vi "OCR Training Tool.vi"() -> ()   [LabVIEW 2018, in "Receipt Parsing.lvlib"]
uses:
  Receipt Parsing.lvlib
  <vilib>/vision/OCR.llb/IMAQ OCR Character Report 2.ctl
  <vilib>/vision/NI_Vision_Development_Module.lvlib
panel:
  out "spreadsheet string":string
  out "Number of Objects":i32
  out "Image 2":T1(plugin-control)
  in  "Min height":i32=450
  out "height (pixels)":i32
  out "width (pixels)":i32
  in  "Submit":bool
  in  "Skip":bool
  in  "Quit":bool
  in  "Character":string
  in  "Min classification score":i32=450
  out "Read String":string
  out "Character Reports":T2[](array[typedef]) {"Character Statistics"."Threshold Range"."Upper value" format="%.2f"; "Character Statistics"."Threshold Range"."Lower value" format="%.2f"}
  out "selected path":path
  out "Post-trained Read":string
  out "Pre-trained Read":string
  out "Image":T1(plugin-control)
  # "Overview: Demonstrates how to train characters to an OCR and compare the readings. \nRequirements: LabVIEW Base Development System 2012 (or compatible)\n                             NI Vision Development Module 2012 (or compatible)\nInstructions: \n1. Run the VI."
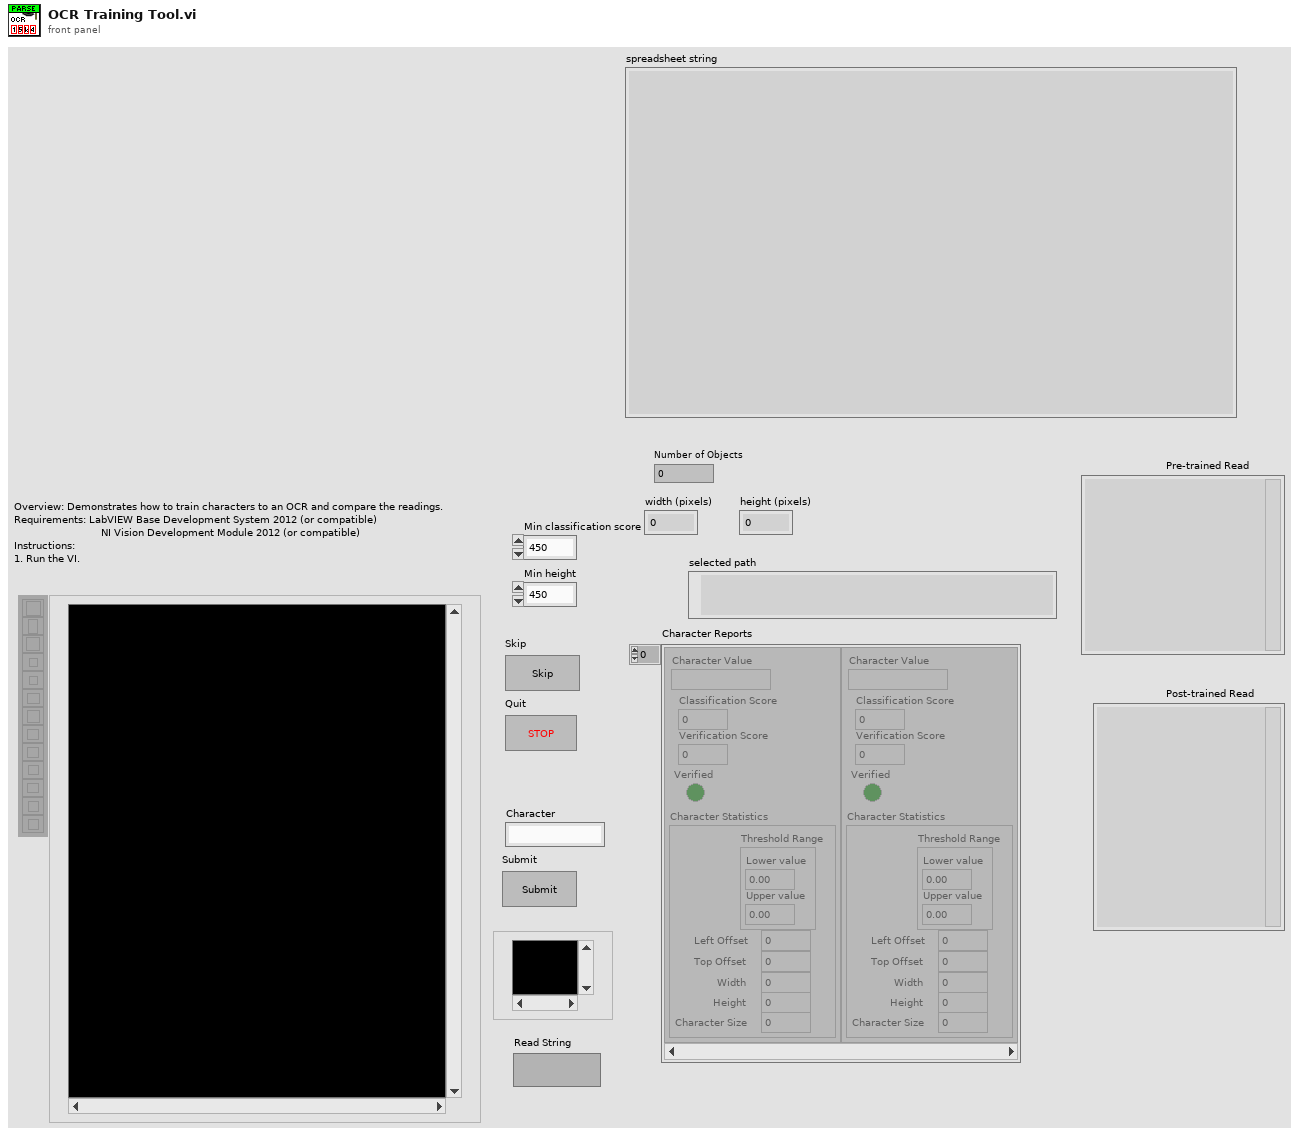
[diagram p1: front panel]
types:
  T1 = typedef "IMAQ Image.ctl" = refnum<image>
  T2 = typedef "IMAQ OCR Character Report 2.ctl" = cluster{"Character Value":string, "Classification Score":i32, "Verification Score":i32, "Verified":bool, "Character Statistics":cluster{"Threshold Range":cluster{"Lower value":sgl, "Upper value":sgl}, "Left Offset":i32, "Top Offset":i32, "Width":i32, "Height":i32, "Character Size":i32}}
  T3 = cluster{"Objects":u16, "Threshold":i32, "Reject Border":bool, "Fill Holes":bool, "Min Object Size":bool, "Min Size":i32, "Max Object Size":bool, "Max Size":i32, "Show Search Area":bool, "Show Center":bool, "Show Bounding Box":bool}
  T4 = typedef "IMAQ OCR Session.ctl" = refnum<k1>
  T5 = typedef "IMAQ Rectangle" = cluster{"Left":i32, "Top":i32, "Right":i32, "Bottom":i32, "Rotation":dbl}
  T6 = cluster{"Object Center":cluster{"X":sgl, "Y":sgl}, "Bounding Box":cluster{"X Left":i32, "Y Top":i32, "X Right":i32, "Y Bottom":i32}, "Area":sgl, "Orientation":sgl, "Aspect Ratio":sgl, "Nb Holes":i32}[]
  T7 = cluster{"X Left":i32, "Y Top":i32, "X Right":i32, "Y Bottom":i32}
  T8 = typedef "ROI Descriptor" = cluster{"Global Rectangle":i32[], "Contours":cluster{"ID":enum32{"External", "Internal"}, "Type":u32, "Coordinates":i32[]}[]}
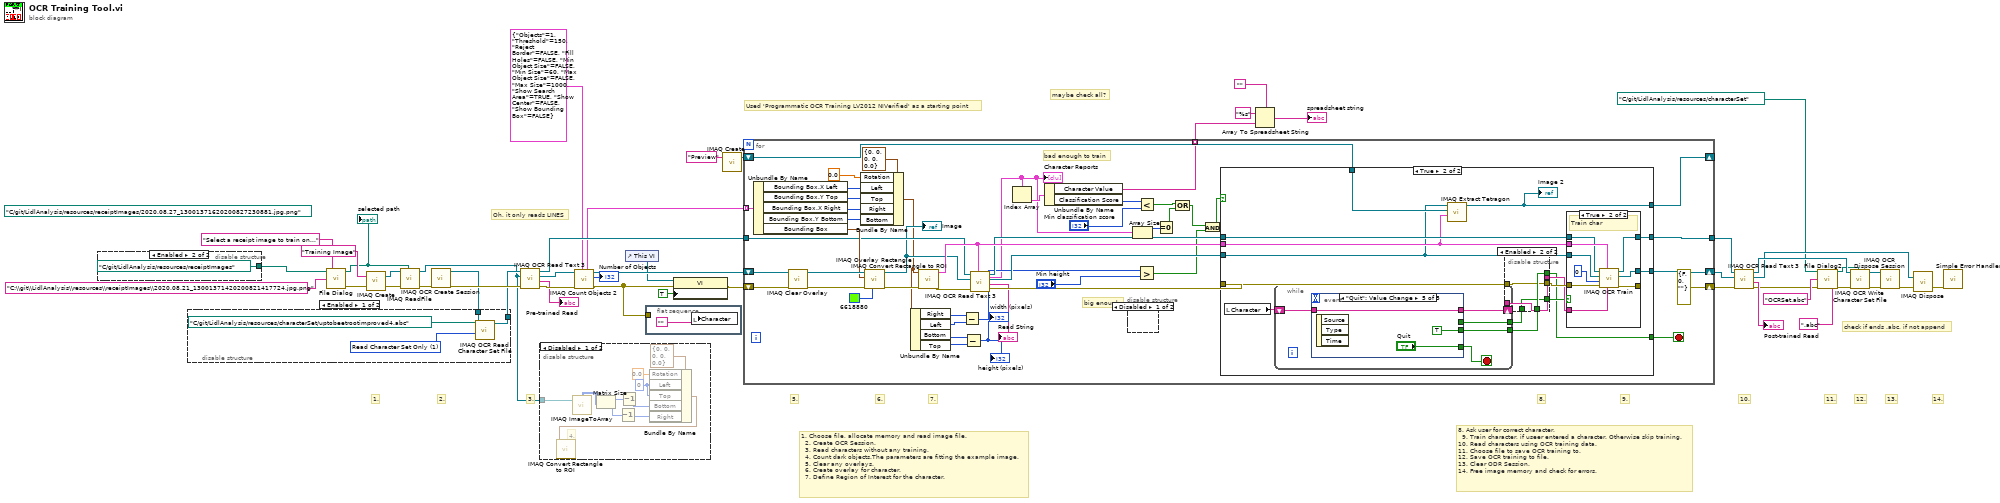
[diagram p0: block diagram]
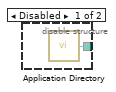
[diagram p3: hidden frame]
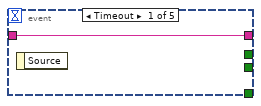
[diagram p7: hidden frame]
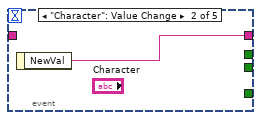
[diagram p8: hidden frame]
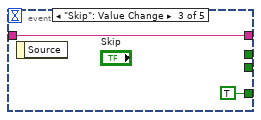
[diagram p9: hidden frame]
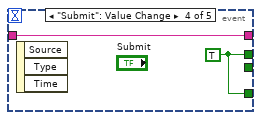
[diagram p10: hidden frame]
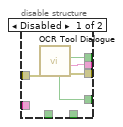
[diagram p11: hidden frame]
diagram:
  (unwired) path "C:/git/LidlAnalysis/resources/receiptImages/2020.08.27_13001371620200827230881.jpg.png" ("File Path")
  # "Oh, it only reads LINES"
  # "maybe check all?"
  # "check if ends .abc, if not append"
  # "Used 'Programmatic OCR Training LV2012 NIVerified' as a starting point"
  # "8. Ask user for correct character.\n  9. Train character, if useer entered a character. Otherwise skip training.\n10. Read characters using OCR training data.\n11. Choose file to save OCR training to.\n12. Save OCR training to file.\n13. Clear ODR Session.\n14. Free image memory and check for errors."
  # "1. Choose file, allocate memory and read image file.\n  2. Create OCR Session.\n  3. Read characters without any training.\n  4. Count dark objects.The parameters are fitting the example image.\n  5. Clear any overlays.\n  6. Create overlay for character.\n  7. Define Region of Interest for the character."
  # "14."
  # "13."
  # "12."
  # "11."
  # "10."
  # "9."
  # "8."
  # "7."
  # "6."
  # "5."
  # "3."
  # "2."
  # "1."
  n1 = disable-structure shown="Enabled" {
    disable-tunnel: [w48 path "C:/git/LidlAnalysis/resources/receiptImages" ("start path")] -> w29
    frame Disabled {
      n2 = call <vilib>:"Application Directory.vi"() -> ("Application Directory"=w48:path)
    }
    frame Enabled {
    }
  }
  n3 = call "File Dialog"("start path"=w29, "prompt"="Select a receipt image to train on...", "default name"="C:\\git\\LidlAnalysis\\resources\\receiptImages\\2020.08.21_13001371420200821417724.jpg.png") -> ("selected path"=w26:path, "error out"=w27:errorcluster)  [unwired: 9 in, 2 out]
  "selected path" <- w26
  n4 = call "IMAQ Create"("Image Name"="Training Image", "error in (no error)"=w27) -> ("New Image"=w46:T1, "error out"=w44:errorcluster)  [unwired: 3 in]
  n5 = call "IMAQ ReadFile"("File Path"=w26, "error in (no error)"=w44, "Image"=w46) -> ("error out"=w43:errorcluster, "Image Out"=w10:T1)  [unwired: 4 in, 3 out]
  n6 = call "IMAQ OCR Create Session"("error in (no error)"=w43) -> ("error out"=w39:errorcluster, "IMAQ OCR Session"=w20:T4)  [unwired: 9 in]
  n7 = disable-structure shown="Enabled" {
    disable-tunnel: w20 -> [w52 w54]
    disable-tunnel: [w51 w54] -> w19
    frame Enabled {
      w53 = 1 items=["Read All", "Read Character Set Only", "Read Properties Only"] ("Read Options")
      n8 = call "IMAQ OCR Read Character Set File"("File Path"=path "C:/git/LidlAnalysis/resources/characterSet/uptobeetrootimproved4.abc", "Read Options"=w53, "IMAQ OCR Session"=w52) -> ("IMAQ OCR Session (dup)"=w51:T4)  [unwired: 6 in, 2 out]
    }
    frame Disabled {
    }
  }
  n9 = call "IMAQ OCR Read Text 3"("error in (no error)"=w39, "Image"=w10, "IMAQ OCR Session"=w19) -> ("error out"=w47:errorcluster, "Read String"=→"Pre-trained Read":string, "Image (dup)"=w11:T1, "IMAQ OCR Session (dup)"=w40:T4)  [unwired: 3 in, 2 out]
  n10 = disable-structure shown="Disabled" {
    disable-tunnel: w10 -> [w60 _]
    frame Disabled {
      w62 = 0 ("Left")
      # "4."
      n11 = call "IMAQ ImageToArray"("Image"=w60) -> ("Image Pixels (U8)"=w64:u8[][])  [unwired: 3 in, 4 out]
      n12 = Matrix Size(0:w64) -> (1:w58:i32, 2:w55:i32)
      n13 = Decrement(x=w55) -> (x-1=w56:i32)
      n14 = Decrement(x=w58) -> (x-1=w57:i32)
      n15 = Bundle By Name(cluster=T5 {"Left"=0, "Top"=0, "Right"=0, "Bottom"=0, "Rotation"=0.0} ("Rectangle"), "Rotation"=0.0, "Left"=w62, "Top"=w62, "Bottom"=w57, "Right"=w56) -> (w61:T5)
      n16 = call "IMAQ Convert Rectangle to ROI"("Rectangle"=w61) -> ()  [unwired: 8 in, 2 out]
    }
    frame Enabled {
    }
  }
  n17 = call "IMAQ Count Objects 2"("Settings"=T3 {"Objects"=1, "Threshold"=150, "Reject Border"=FALSE, "Fill Holes"=FALSE, "Min Object Size"=FALSE, "Min Size"=60, "Max Object Size"=FALSE, "Max Size"=1000, "Show Search Area"=TRUE, "Show Center"=FALSE, "Show Bounding Box"=FALSE}, "error in (no error)"=w47, "Image"=w11) -> ("error out"=w1:errorcluster, "Number of Objects"=→"Number of Objects":i32, "Image Out"=w34:T1, "Objects"=w33:T6)  [unwired: 4 in, 1 out]
  n18 = control-ref of="This VI"() -> (w14:refnum<vi>)
  n19 = flat-sequence {
    tunnel: w1 -> [_]
    frame #0 {
      n20 = local write "Character"("") -> ()
    }
  }
  n21 = property class="VI"(reference=w14, error in=w1, "Front Panel.IsFrontmost"=TRUE ("Front Panel Window:Is Frontmost")) -> (error out=w13:errorcluster)  [unwired: 1 out]
  n22 = call "IMAQ Create"("Image Name"="Preview") -> ("New Image"=w8:T1)  [unwired: 4 in, 1 out]
  n23 = for {
    shift-right: [errorcluster {"status"=FALSE, "code"=0, "source"=""} ("error out")] -> w35
    shift-left: w13 -> [w112]
    shift-right: [w111] -> w17
    shift-left: w34 -> [w108]
    tunnel: w33 -> [w106] mode=indexing
    tunnel: w40 -> [w90]
    tunnel: [w110] -> w18
    shift-right: [w74] -> _
    shift-left: w8 -> [w73]
    tunnel: [w66] -> w5 mode=indexing
    stop <- w95 stop-if-true
    # "bad enough to train"
    # "big enough"
    n24 = Unbundle By Name(w106) -> ("Bounding Box.X Left"=w101:i32, "Bounding Box.Y Top"=w100:i32, "Bounding Box.X Right"=w99:i32, "Bounding Box.Y Bottom"=w98:i32, "Bounding Box"=w105:T7)
    n25 = call "IMAQ Clear Overlay"("error in (no error)"=w112, "Image"=w108) -> ("error out"=w109:errorcluster, "Image Out"=w107:T1)  [unwired: 8 in]
    n26 = Bundle By Name(cluster=T5 {"Left"=0, "Top"=0, "Right"=0, "Bottom"=0, "Rotation"=0.0} ("Rectangle"), "Rotation"=0.0, "Left"=w101, "Top"=w100, "Right"=w99, "Bottom"=w98) -> (w83:T5)
    n27 = call "IMAQ Overlay Rectangle"("Color"=u32 6618880, "error in (no error)"=w109, "Rectangle"=w105, "Image"=w107) -> ("error out"=w103:errorcluster, "Image Out"=w89:T1)  [unwired: 6 in]
    "Image" <- w89
    n28 = Unbundle By Name(w83) -> ("Right"=w82:i32, "Left"=w81:i32, "Bottom"=w80:i32, "Top"=w79:i32)
    n29 = call "IMAQ Convert Rectangle to ROI"("error in (no error)"=w103, "Rectangle"=w83) -> ("error out"=w94:errorcluster, "ROI Descriptor"=w92:T8)  [unwired: 7 in]
    n30 = Subtract(x=w82, y=w81) -> (x-y=→"width (pixels)":i32)
    n31 = Subtract(x=w80, y=w79) -> (x-y=w75:i32)
    "height (pixels)" <- w75
    n32 = call "IMAQ OCR Read Text 3"("ROI Descriptor"=w92, "error in (no error)"=w94, "Image"=w89, "IMAQ OCR Session"=w90) -> ("error out"=w93:errorcluster, "Read String"=→"Read String":string, "Image (dup)"=w88:T1, "IMAQ OCR Session (dup)"=w91:T4, "Character Reports"=w72:T2[])  [unwired: 2 in, 1 out]
    "Character Reports" <- w72
    n33 = Index Array(array=w72) -> (element=w86:T2)  [unwired: 1 in]
    n34 = Unbundle By Name(w86) -> ("Character Value"=w66:string, "Classification Score"=w85:i32)
    n35 = disable-structure shown="Disabled" {
      frame Disabled {
      }
      frame Enabled {
      }
    }
    n36 = Array Size(array=w72) -> (size(s)=w71:i32)
    n37 = Greater?(x=w75, y="Min height") -> (0:w69:bool)
    n38 = Less?(x=w85, y="Min classification score") -> (x < y?=w77:bool)
    n39 = Equal To 0?(x=w71) -> (x = 0?=w70:bool)
    n40 = Compound Arithmetic op=OR(w77, w70) -> (w68:bool)
    n41 = And(x=w68, y=w69) -> (x .and. y?=w67:bool)
    n42 = case shown="True" w67 {
      tunnel: [w115 w131] -> w111
      tunnel: [w114 w130] -> w110
      tunnel: [_ w126] -> w95
      tunnel: w93 -> [_ w124]
      tunnel: w92 -> [_ w119]
      tunnel: w91 -> [w114 w125]
      tunnel: w88 -> [w115 w118]
      tunnel: w73 -> [w113 w120]
      tunnel: [w113 w117] -> w74
      frame False {
        # "No need to train"
      }
      frame True {
        n43 = local read "Character"() -> (w116:string)
        n44 = while {
          tunnel: [w135] -> w123
          tunnel: [w134] -> w121
          shift-right: [w133] -> w122
          shift-left: w116 -> [w132]
          stop <- w136 stop-if-true
          n45 = event shown="[4] \"Quit\": Value Change" {
            selector: _ -> [_ _ _ _ _]
            dyn-events: _ -> [_ _ _ _ _]
            timeout: _ -> [_ _ _ _ _]
            tunnel: [_ _ TRUE ("Quit") w142 "Quit"] -> w136
            tunnel: [_ _ _ _ TRUE] -> w135
            tunnel: [_ _ _ w142 _] -> w134
            tunnel: [w137 w138 w139 w141 w143] -> w133
            tunnel: w132 -> [w137 _ w139 w141 w143]
            event Timeout {
              n46 = event-data() -> ()  [unwired: 1 in, 1 out]
            }
            event "Character": Value Change {
              n47 = event-data() -> ("NewVal"=w138:string)  [unwired: 1 in]
            }
            event "Skip": Value Change {
              n48 = event-data() -> ()  [unwired: 1 in, 1 out]
            }
            event "Submit": Value Change {
              w142 = TRUE
              n49 = event-data() -> ()  [unwired: 1 in, 3 out]
            }
            event "Quit": Value Change {
              n50 = event-data() -> ()  [unwired: 1 in, 3 out]
            }
          }
        }
        n51 = call-poly "IMAQ Extract Tetragon"("ROI Descriptor"=w119, "Image Dst"=w120, "Image Src"=w118) -> ("Image Dst Out"=w117:T1)  [unwired: 7 in, 1 out]
        "Image 2" <- w117
        n52 = disable-structure shown="Enabled" {
          disable-tunnel: [w150 w152] -> w129
          disable-tunnel: [w149 w153] -> w128
          disable-tunnel: [w148 w151] -> w127
          disable-tunnel: w124 -> [w147 w152]
          disable-tunnel: [w146 w154] -> w126
          disable-tunnel: w123 -> [_ w154]
          disable-tunnel: w122 -> [_ w153]
          disable-tunnel: w121 -> [_ w151]
          frame Disabled {
            n53 = call "OCR Tool Dialogue.vi"("error in (no error)"=w147) -> ("error out"=w150:errorcluster, "Character"=w149:string, "Quitted?"=w146:bool, "Enter Char"=w148:bool)  [unwired: 7 in]
          }
          frame Enabled {
          }
        }
        n54 = case shown="True" w127 {
          tunnel: [w156 w165] -> w131
          tunnel: [w157 w164] -> _
          tunnel: w125 -> [w155 w163]
          tunnel: [w155 w162] -> w130
          tunnel: w118 -> [w156 w161]
          tunnel: w129 -> [w157 w160]
          tunnel: w128 -> [_ w159]
          tunnel: w119 -> [_ w166]
          frame False {
            # "User input: not a char"
          }
          frame True {
            # "Train char"
            n55 = call "IMAQ OCR Train"("Character Value"=w159, "ROI Descriptor"=w166, "error in (no error)"=w160, "Object Index"=0, "Image"=w161, "IMAQ OCR Session"=w163) -> ("error out"=w164:errorcluster, "Image (dup)"=w165:T1, "IMAQ OCR Session (dup)"=w162:T4)  [unwired: 3 in]
          }
        }
      }
    }
  }
  n56 = Array To Spreadsheet String(delimiter (Tab)="", array=w5, 3:"%s" ("format string")) -> (spreadsheet string=→"spreadsheet string":string)
  n57 = call "IMAQ OCR Read Text 3"("error in (no error)"=w35, "Image"=w17, "IMAQ OCR Session"=w18) -> ("error out"=w23:errorcluster, "Read String"=→"Post-trained Read":string, "Image (dup)"=w30:T1, "IMAQ OCR Session (dup)"=w37:T4)  [unwired: 3 in, 2 out]
  n58 = call "File Dialog2"("start path"=path "C:/git/LidlAnalysis/resources/characterSet", "default name"="OCRSet.abc" ("name or relative path"), "error in"=w23, "pattern label"=".abc") -> ("selected path"=w21:path, "error out"=w24:errorcluster)  [unwired: 8 in, 2 out]
  n59 = call "IMAQ OCR Write Character Set File"("File Path"=w21, "error in (no error)"=w24, "IMAQ OCR Session"=w37) -> ("error out"=w42:errorcluster, "IMAQ OCR Session (dup)"=w41:T4)  [unwired: 7 in]
  n60 = call "IMAQ OCR Dispose Session"("error in (no error)"=w42, "IMAQ OCR Session"=w41) -> ("error out"=w22:errorcluster)  [unwired: 9 in]
  n61 = call "IMAQ Dispose"("Image"=w30, "error in (no error)"=w22) -> ("error out"=w31:errorcluster)  [unwired: 4 in]
  n62 = call <vilib>:"Simple Error Handler.vi"("error in (no error)"=w31) -> ()  [unwired: 4 in, 5 out]
